vi "SN Generating_VNA.vi"(5 "Start":bool, 7 "Sart SN":i32=3000, 8 "Product Type":string(combo)="SFP+") -> (0 "note":string="T", 1 "show_int_XXXX":i32, 2 "show_int_yydddXXXX":i32, 3 "Initial SN":i32=153100000)   [LabVIEW 2011]
uses:
  <vilib>/addons/database/NI_Database_API.lvlib
  <vilib>/addons/database/Connection.llb/DB Tools Open Connec (String).vi
  <vilib>/addons/database/_DB Variant To Data/Database Variant To Data.xnode
panel:
  in  "Product Type 2":string(combo)="SFP+"
  out "SN 2":string="12V"
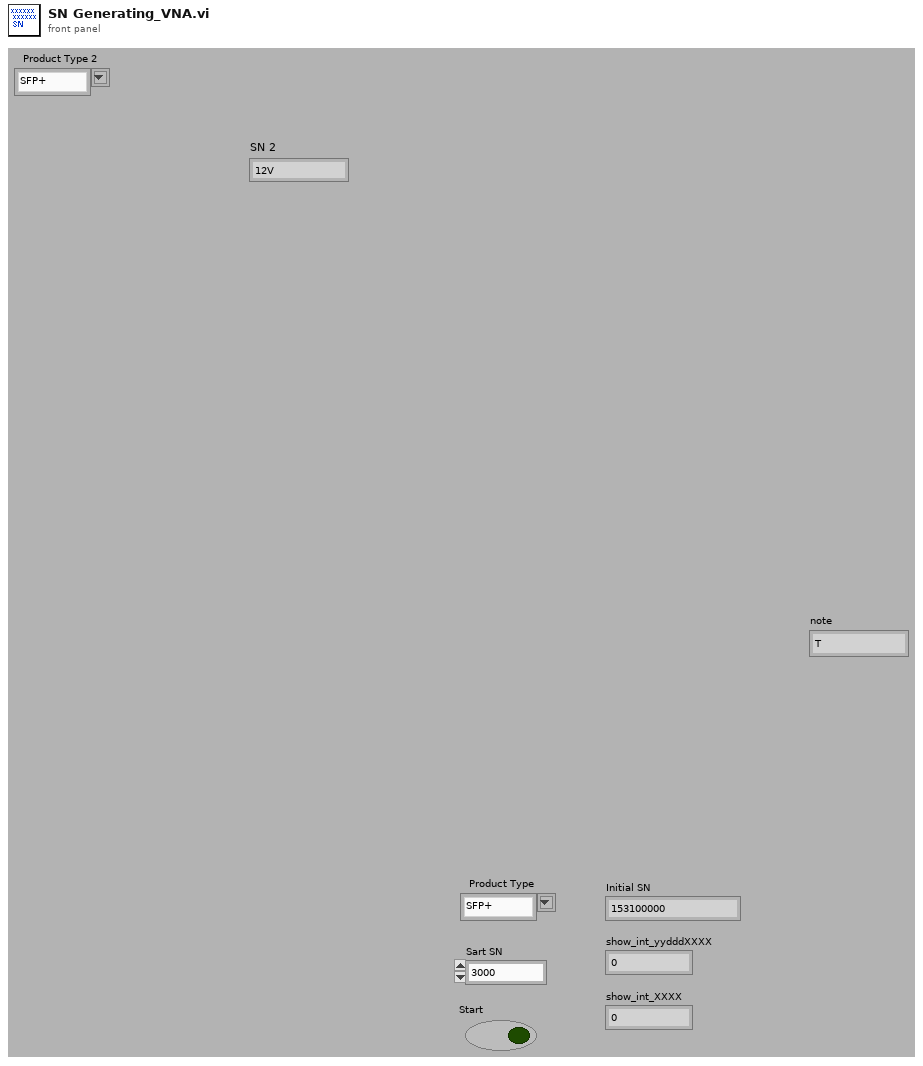
[diagram p1: front panel]
types:
  T1 = typedef "NI_Database_API.lvlib/Conn ObjectReference.ctl" = refnum<k1>
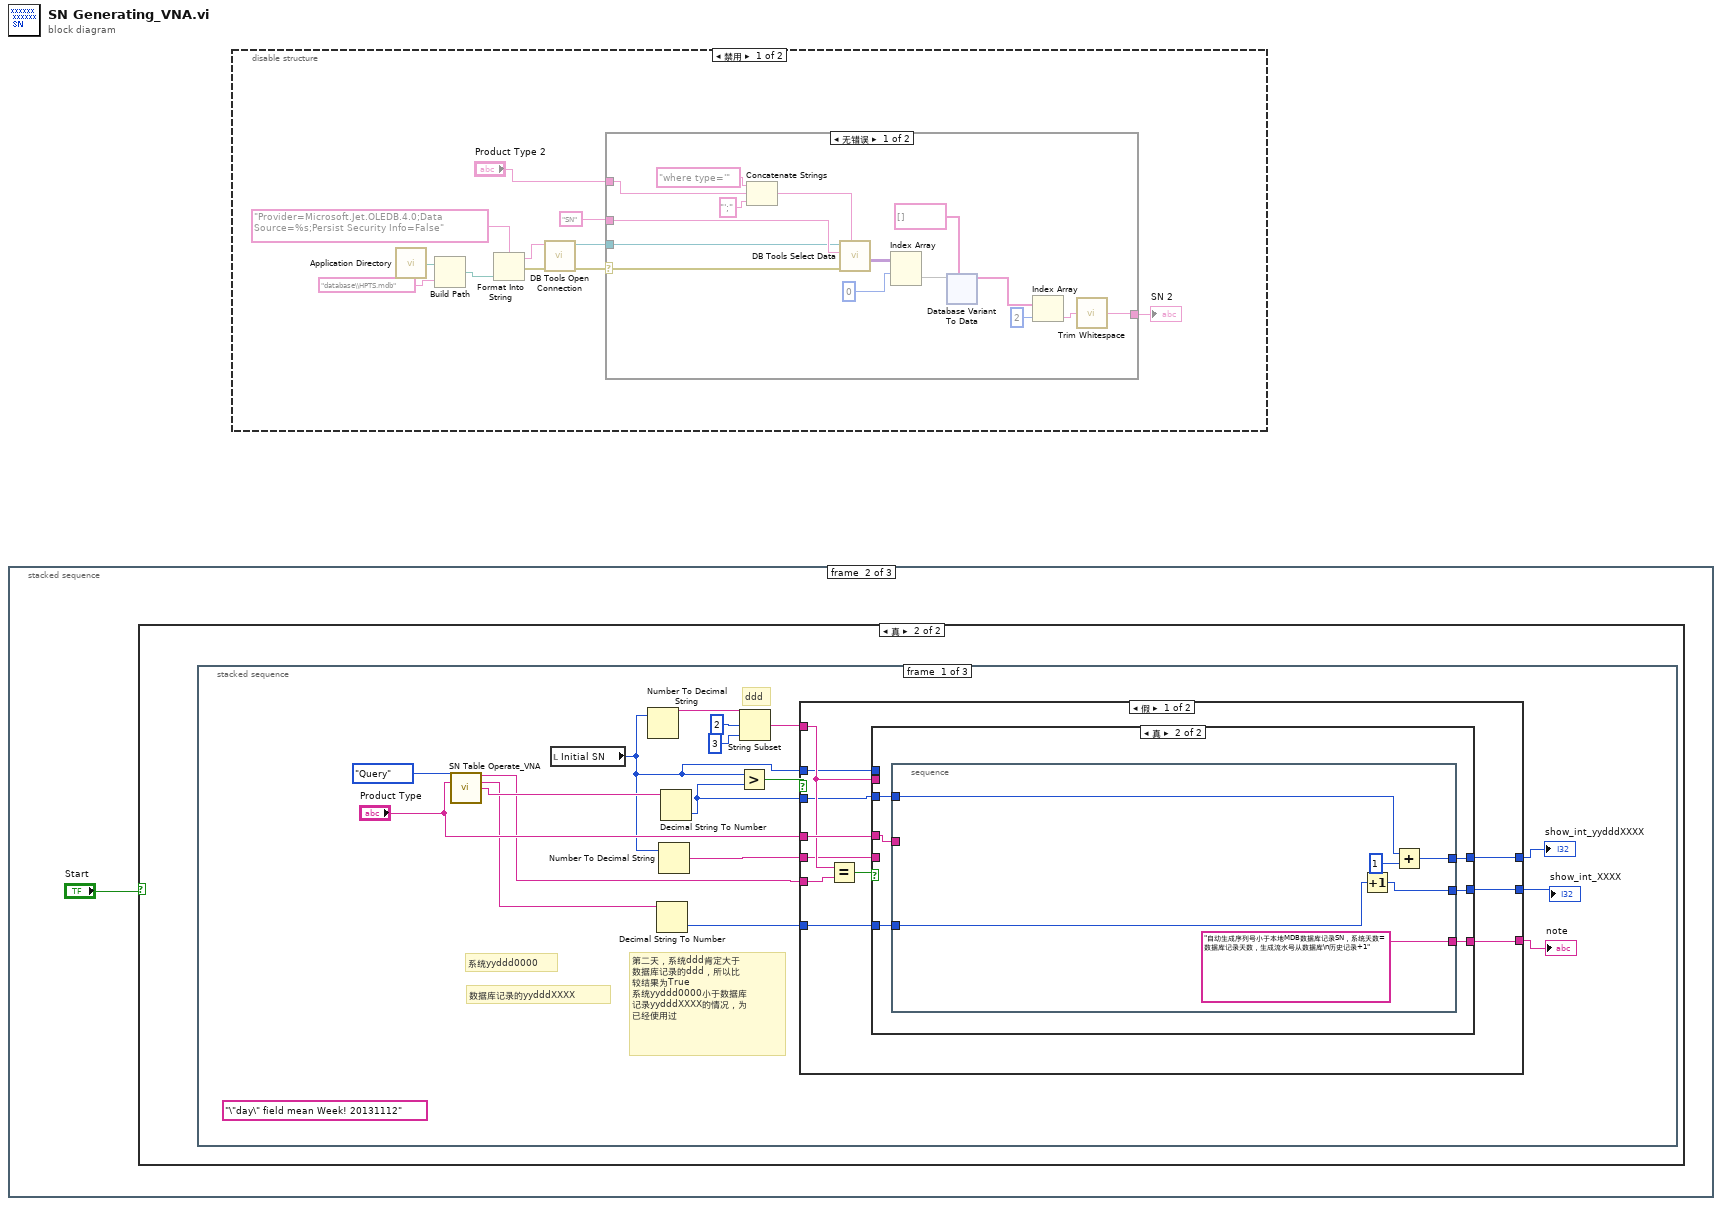
[diagram p0: block diagram]
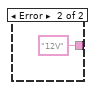
[diagram p2: hidden frame]
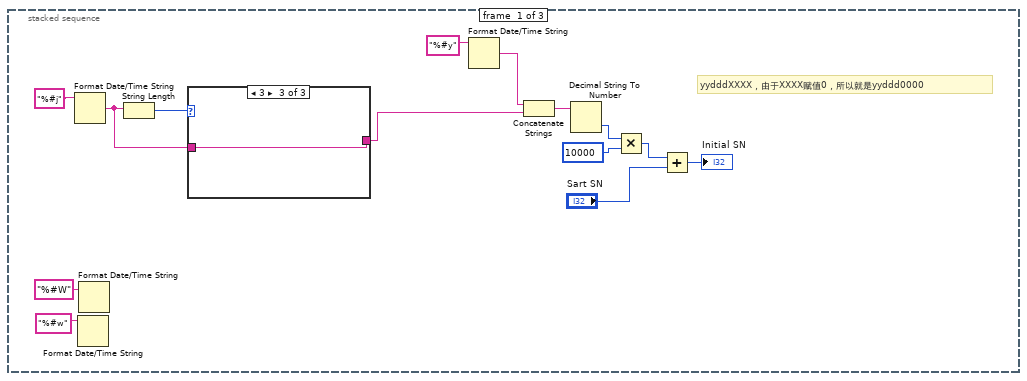
[diagram p4: hidden frame]
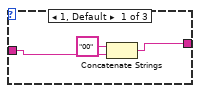
[diagram p5: hidden frame]
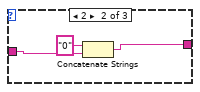
[diagram p6: hidden frame]
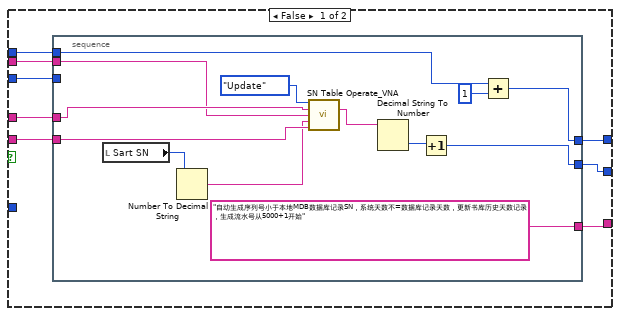
[diagram p8: hidden frame]
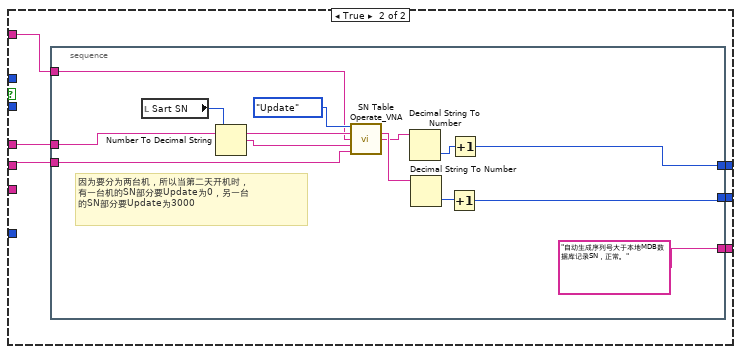
[diagram p9: hidden frame]
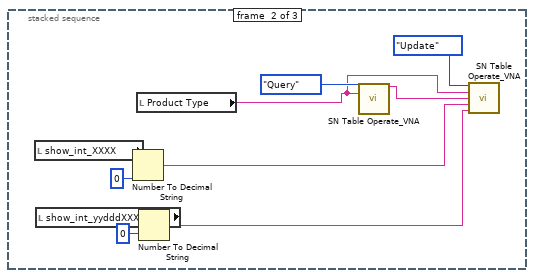
[diagram p10: hidden frame]
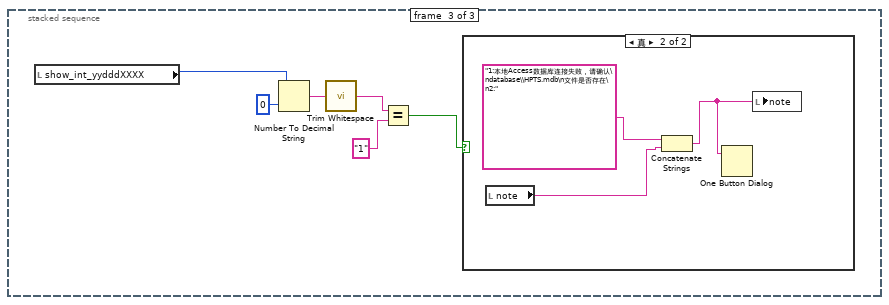
[diagram p11: hidden frame]
diagram:
  n1 = stacked-sequence {
    frame #0 {
      # "yydddXXXX，由于XXXX赋值0，所以就是yyddd0000"
      n2 = Format Date/Time String(time format string (%c)="%#j") -> (date/time string=w2:string)  [unwired: 2 in]
      n3 = Format Date/Time String(time format string (%c)="%#w") -> ()  [unwired: 2 in, 1 out]
      n4 = Format Date/Time String(time format string (%c)="%#W") -> ()  [unwired: 2 in, 1 out]
      n5 = String Length(string=w2) -> (length=w3:i32)
      n6 = case shown="3" w3 {
        tunnel: w2 -> [w16 w20 w21]
        tunnel: [w15 w19 w21] -> w1
        frame 1, Default {
          n7 = Concatenate Strings("00" ("字符串"), w16) -> (w15:string)
        }
        frame 2 {
          n8 = Concatenate Strings("0" ("字符串"), w20) -> (w19:string)
        }
        frame 3 {
        }
      }
      n9 = Format Date/Time String(time format string (%c)="%#y") -> (date/time string=w14:string)  [unwired: 2 in]
      n10 = Concatenate Strings(w14, w1) -> (w12:string)
      n11 = Decimal String To Number(string=w12) -> (number=w11:i32)  [unwired: 2 in, 1 out]
      n12 = Multiply(x=w11, y=10000) -> (x*y=w8:i32)
      n13 = Add(x=w8, y="Sart SN") -> (x+y=→"Initial SN":i32)
    }
    frame #1 {
      n14 = case shown="真" "Start" {
        frame False {
        }
        frame True {
          n15 = stacked-sequence {
            frame #0 {
              (unwired) "\"day\" field mean Week! 20131112" ("Command Text")
              # "第二天，系统ddd肯定大于\n数据库记录的ddd，所以比\n较结果为True\n系统yyddd0000小于数据库\n记录yydddXXXX的情况，为\n已经使用过"
              # "数据库记录的yydddXXXX"
              # "系统yyddd0000"
              # "ddd"
              n16 = call "SN Table Operate_VNA.vi"("Function"=enum16{"Query", "Update"}."Query", "Product Type"="Product Type") -> ("Day"=w29:string, "Tail"=w27:string, "SN_OUT"=w30:string)  [unwired: 11 in]
              n17 = local read "Initial SN"() -> (w24:i32)
              n18 = Number To Decimal String(number=w24) -> (decimal integer string=w36:string)  [unwired: 1 in]
              n19 = Decimal String To Number(string=w27) -> (number=w26:i32)  [unwired: 2 in, 1 out]
              n20 = Number To Decimal String(number=w24) -> (decimal integer string=w28:string)  [unwired: 1 in]
              n21 = Decimal String To Number(string=w30) -> (number=w25:i32)  [unwired: 2 in, 1 out]
              n22 = Greater?(x=w24, y=w25) -> (0:w39:bool)
              n23 = String Subset(string=w36, offset (0)=2 ("偏移量(0)"), length (rest)=3 ("长度（剩余）")) -> (substring=w33:string)
              n24 = case shown="假" w39 {
                tunnel: "Product Type" -> [w50 w89]
                tunnel: [w49 w88] -> w38
                tunnel: [w48 w87] -> w37
                tunnel: w33 -> [w45 w86]
                tunnel: w29 -> [w47 _]
                tunnel: w28 -> [w42 w85]
                tunnel: w26 -> [w43 _]
                tunnel: w25 -> [w44 _]
                tunnel: w24 -> [w41 _]
                tunnel: [w40 w84] -> w23
                frame False {
                  n25 = Equal?(x=w45, y=w47) -> (x = y?=w46:bool)
                  n26 = case shown="真" w46 {
                    tunnel: w50 -> [w57 w77]
                    tunnel: w44 -> [w54 w76]
                    tunnel: [w55 w75] -> w49
                    tunnel: [w56 w74] -> w48
                    tunnel: w45 -> [w58 _]
                    tunnel: w43 -> [_ w73]
                    tunnel: w42 -> [w53 _]
                    tunnel: w41 -> [w52 _]
                    tunnel: [w51 w72] -> w40
                    frame False {
                      n27 = stacked-sequence {
                        tunnel: w58 -> [w69]
                        tunnel: w57 -> [w70]
                        tunnel: [w64] -> w56
                        tunnel: [w65] -> w55
                        tunnel: w54 -> [_]
                        tunnel: w53 -> [w68]
                        tunnel: w52 -> [w66]
                        tunnel: ["自动生成序列号小于本地MDB数据库记录SN，系统天数不=数据库记录天数，更新书库历史天数记录，生成流水号从5000+1开始"] -> w51
                        frame #0 {
                          n28 = local read "Sart SN"() -> (w60:i32)
                          n29 = Number To Decimal String(number=w60) -> (decimal integer string=w59:string)  [unwired: 1 in]
                          n30 = call "SN Table Operate_VNA.vi"("Function"=enum16{"Query", "Update"}."Update", "Product Type"=w70, "Day in"=w69, "Tail in"=w59, "SN In"=w68) -> ("Tail"=w63:string)  [unwired: 8 in, 2 out]
                          n31 = Decimal String To Number(string=w63) -> (number=w67:i32)  [unwired: 2 in, 1 out]
                          n32 = Increment(x=w67) -> (x+1=w64:i32)
                          n33 = Add(x=w66, y=1) -> (x+y=w65:i32)
                        }
                      }
                    }
                    frame True {
                      n34 = stacked-sequence {
                        tunnel: w77 -> [_]
                        tunnel: w76 -> [w83]
                        tunnel: [w82] -> w75
                        tunnel: [w81] -> w74
                        tunnel: w73 -> [w80]
                        tunnel: ["自动生成序列号小于本地MDB数据库记录SN，系统天数=数据库记录天数，生成流水号从数据库\n历史记录+1"] -> w72
                        frame #0 {
                          n35 = Increment(x=w80) -> (x+1=w81:i32)
                          n36 = Add(x=w83, y=1) -> (x+y=w82:i32)
                        }
                      }
                    }
                  }
                }
                frame True {
                  n37 = stacked-sequence {
                    tunnel: w89 -> [w102]
                    tunnel: [w94] -> w88
                    tunnel: [w97] -> w87
                    tunnel: w86 -> [w100]
                    tunnel: w85 -> [w93]
                    tunnel: ["自动生成序列号大于本地MDB数据库记录SN，正常。"] -> w84
                    frame #0 {
                      # "因为要分为两台机，所以当第二天开机时，\n有一台机的SN部分要Update为0，另一台\n的SN部分要Update为3000"
                      n38 = local read "Sart SN"() -> (w91:i32)
                      n39 = Number To Decimal String(number=w91) -> (decimal integer string=w90:string)  [unwired: 1 in]
                      n40 = call "SN Table Operate_VNA.vi"("Function"=enum16{"Query", "Update"}."Update", "Product Type"=w102, "Day in"=w100, "Tail in"=w90, "SN In"=w93) -> ("Tail"=w98:string, "SN_OUT"=w96:string)  [unwired: 8 in, 1 out]
                      n41 = Decimal String To Number(string=w96) -> (number=w95:i32)  [unwired: 2 in, 1 out]
                      n42 = Decimal String To Number(string=w98) -> (number=w99:i32)  [unwired: 2 in, 1 out]
                      n43 = Increment(x=w99) -> (x+1=w97:i32)
                      n44 = Increment(x=w95) -> (x+1=w94:i32)
                    }
                  }
                }
              }
              "show_int_yydddXXXX" <- w38
              "show_int_XXXX" <- w37
              "note" <- w23
            }
            frame #1 {
              n45 = local read "show_int_XXXX"() -> (w109:i32)
              n46 = local read "show_int_yydddXXXX"() -> (w110:i32)
              n47 = Number To Decimal String(number=w109, width (-)=i16 0 ("宽度(-)")) -> (decimal integer string=w104:string)
              n48 = local read "Product Type"() -> (w106:string)
              n49 = Number To Decimal String(number=w110, width (-)=i16 0 ("宽度(-)")) -> (decimal integer string=w103:string)
              n50 = call "SN Table Operate_VNA.vi"("Function"=enum16{"Query", "Update"}."Query", "Product Type"=w106) -> ("Day"=w105:string)  [unwired: 11 in, 2 out]
              n51 = call "SN Table Operate_VNA.vi"("Function"=enum16{"Query", "Update"}."Update", "Product Type"=w106, "Day in"=w105, "Tail in"=w104, "SN In"=w103) -> ()  [unwired: 8 in, 3 out]
            }
            frame #2 {
              n52 = local read "show_int_yydddXXXX"() -> (w117:i32)
              n53 = Number To Decimal String(number=w117, width (-)=i16 0 ("宽度(-)")) -> (decimal integer string=w116:string)
              n54 = call <vilib>:"Trim Whitespace.vi"("string"=w116) -> ("trimmed string"=w114:string)  [unwired: 1 in]
              n55 = Equal?(x=w114, y="1") -> (x = y?=w113:bool)
              n56 = case shown="真" w113 {
                frame False {
                }
                frame True {
                  n57 = local read "note"() -> (w120:string)
                  n58 = Concatenate Strings("1:本地Access数据库连接失败，请确认\ndatabase\\HPTS.mdb\n文件是否存在\n2:" ("字符串"), w120) -> (w119:string)
                  n59 = One Button Dialog(message=w119) -> ()  [unwired: 1 in, 1 out]
                  n60 = local write "note"(w119) -> ()
                }
              }
            }
          }
        }
      }
    }
    frame #2 {
    }
  }
  n61 = disable-structure shown="禁用" {
    frame Disabled {
      n62 = call <vilib>:"Application Directory.vi"() -> ("Application Directory"=w132:path)
      n63 = Build Path(base path=w132, name or relative path="database\\HPTS.mdb" ("名称或相对路径")) -> (appended path=w130:path)
      n64 = Format Into String(format string="Provider=Microsoft.Jet.OLEDB.4.0;Data Source=%s;Persist Security Info=False" ("格式字符串"), w130) -> (resulting string=w129:string, error out=w128:errorcluster)  [unwired: 2 in]
      n65 = call-poly <vilib>:"DB Tools Open Connection.vi"("error in (no error)"=w128, "connection information"=w129) -> ("error out"=w126:errorcluster, "connection reference"=w125:T1)  [unwired: 6 in]
      n66 = case shown="无错误" w126 {
        selector: w126 -> [w144 _]
        tunnel: w125 -> [w143 _]
        tunnel: "SN" ("table") -> [w145 _]
        tunnel: [w138 "12V" ("trimmed string")] -> w123
        tunnel: "Product Type 2" -> [w136 _]
        frame No Error {
          n67 = Concatenate Strings("where type='" ("Command Text"), w136, "';" ("字符串")) -> (w134:string)
          n68 = call <vilib>:"DB Tools Select Data.vi"("condition"=w134, "error in (no error)"=w144, "table"=w145, "connection reference"=w143) -> ("data"=w142:variant[][])  [unwired: 2 in, 2 out]
          n69 = Index Array(array=w142, index (row)=0 ("禁用的索引 (列)")) -> (element=w146:variant[])  [unwired: 1 in]
          n70 = xnode "Database Variant To Data"("database variant"=w146, "type"=string[] []) -> ("data"=w141:string[])  [unwired: 1 in, 1 out]
          n71 = Index Array(array=w141, index=2 ("索引")) -> (element=w139:string)
          n72 = call <vilib>:"Trim Whitespace.vi"("string"=w139) -> ("trimmed string"=w138:string)  [unwired: 1 in]
        }
        frame Error {
        }
      }
      "SN 2" <- w123
    }
    frame Enabled {
    }
  }
